vi "Construct Configuration File Binding.vi"(9 "Key Name":string, 10 "Section Name":string, 11 "Config File Refnum":T1) -> (0 "error out":errorcluster, 3 "ConfigurationFileBinding":refnum<class "ConfigurationFileBinding.lvclass">)   [LabVIEW 2017, in "ConfigurationFileBinding.lvclass"]
doc: "<License>\nCopyright © 2017 Composed Systems, LLC | All rights reserved\nwww.composed.io\n\nAuthor: Ethan Stern <ethan.stern@composed.io>\n\nThis software is provided \"AS IS\" WITHOUT WARRANTIES, either express or implied, AND IS FOR EDUCATIONAL PURPOSES ONLY.\n</License>"
uses:
  ConfigurationFileBinding.lvclass
  <vilib>/Utility/config.llb/Config Data RefNum.ctl
  ConfigurationFileBinding.lvclass/ConfigurationFileBinding.ctl
  <vilib>/Utility/error.llb/Error Cluster From Error Code.vi
  <vilib>/ErrorRing/Error Ring.xnode
  <vilib>/Utility/config.llb/NI_LVConfig.lvlib
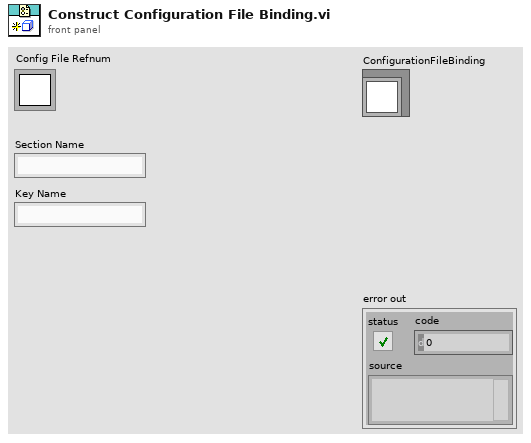
[diagram p1: front panel]
types:
  T1 = typedef "NI_LVConfig.lvlib/Config Data RefNum.ctl" = refnum<k1>
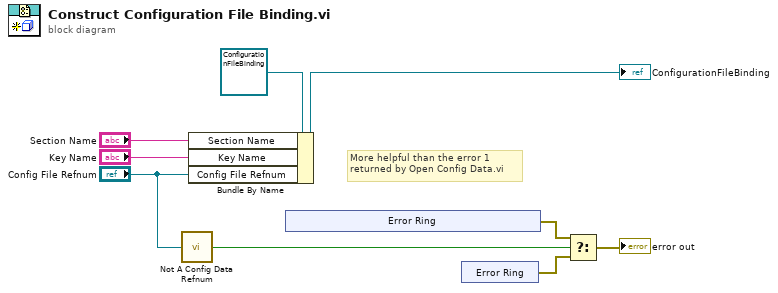
[diagram p0: block diagram]
diagram:
  # "More helpful than the error 1\nreturned by Open Config Data.vi"
  n1 = call <vilib>:"Not A Config Data Refnum.vi"("refnum"="Config File Refnum") -> ("not a config data refnum"=w2:bool)
  n2 = Bundle By Name(cluster=refnum<class "ConfigurationFileBinding.lvclass"> refnum ("ConfigurationFileBinding"), "Section Name"="Section Name", "Key Name"="Key Name", "Config File Refnum"="Config File Refnum") -> (→"ConfigurationFileBinding":refnum<class "ConfigurationFileBinding.lvclass">)
  n3 = xnode "Error Ring"() -> ("error out"=w6:errorcluster)
  n4 = xnode "Error Ring"() -> ("error out"=w5:errorcluster)
  n5 = Select(t=w6, s=w2, f=w5) -> (s? t:f=→"error out":errorcluster)
